vi "DriveStraight4.vi"(7 "Re-Init":bool, 9 "arguments":string[](array[string]), 10 "SensorInputData":T5, 11 "HMI to Control":T1) -> (2 "HMI to Control Out":T1, 3 "SensorInputDataOut":T5, 4 "Done":bool)   [LabVIEW 2015]
uses:
  Typedefs/SensorInputData.ctl
  Typedefs/HMI_to_Control.ctl
  Typedefs/Arm States.ctl
  Typedefs/ClawStates.ctl
  Typedefs/IntakeWheelSenseOrManual.ctl
  scriptlib/auto_data.vi
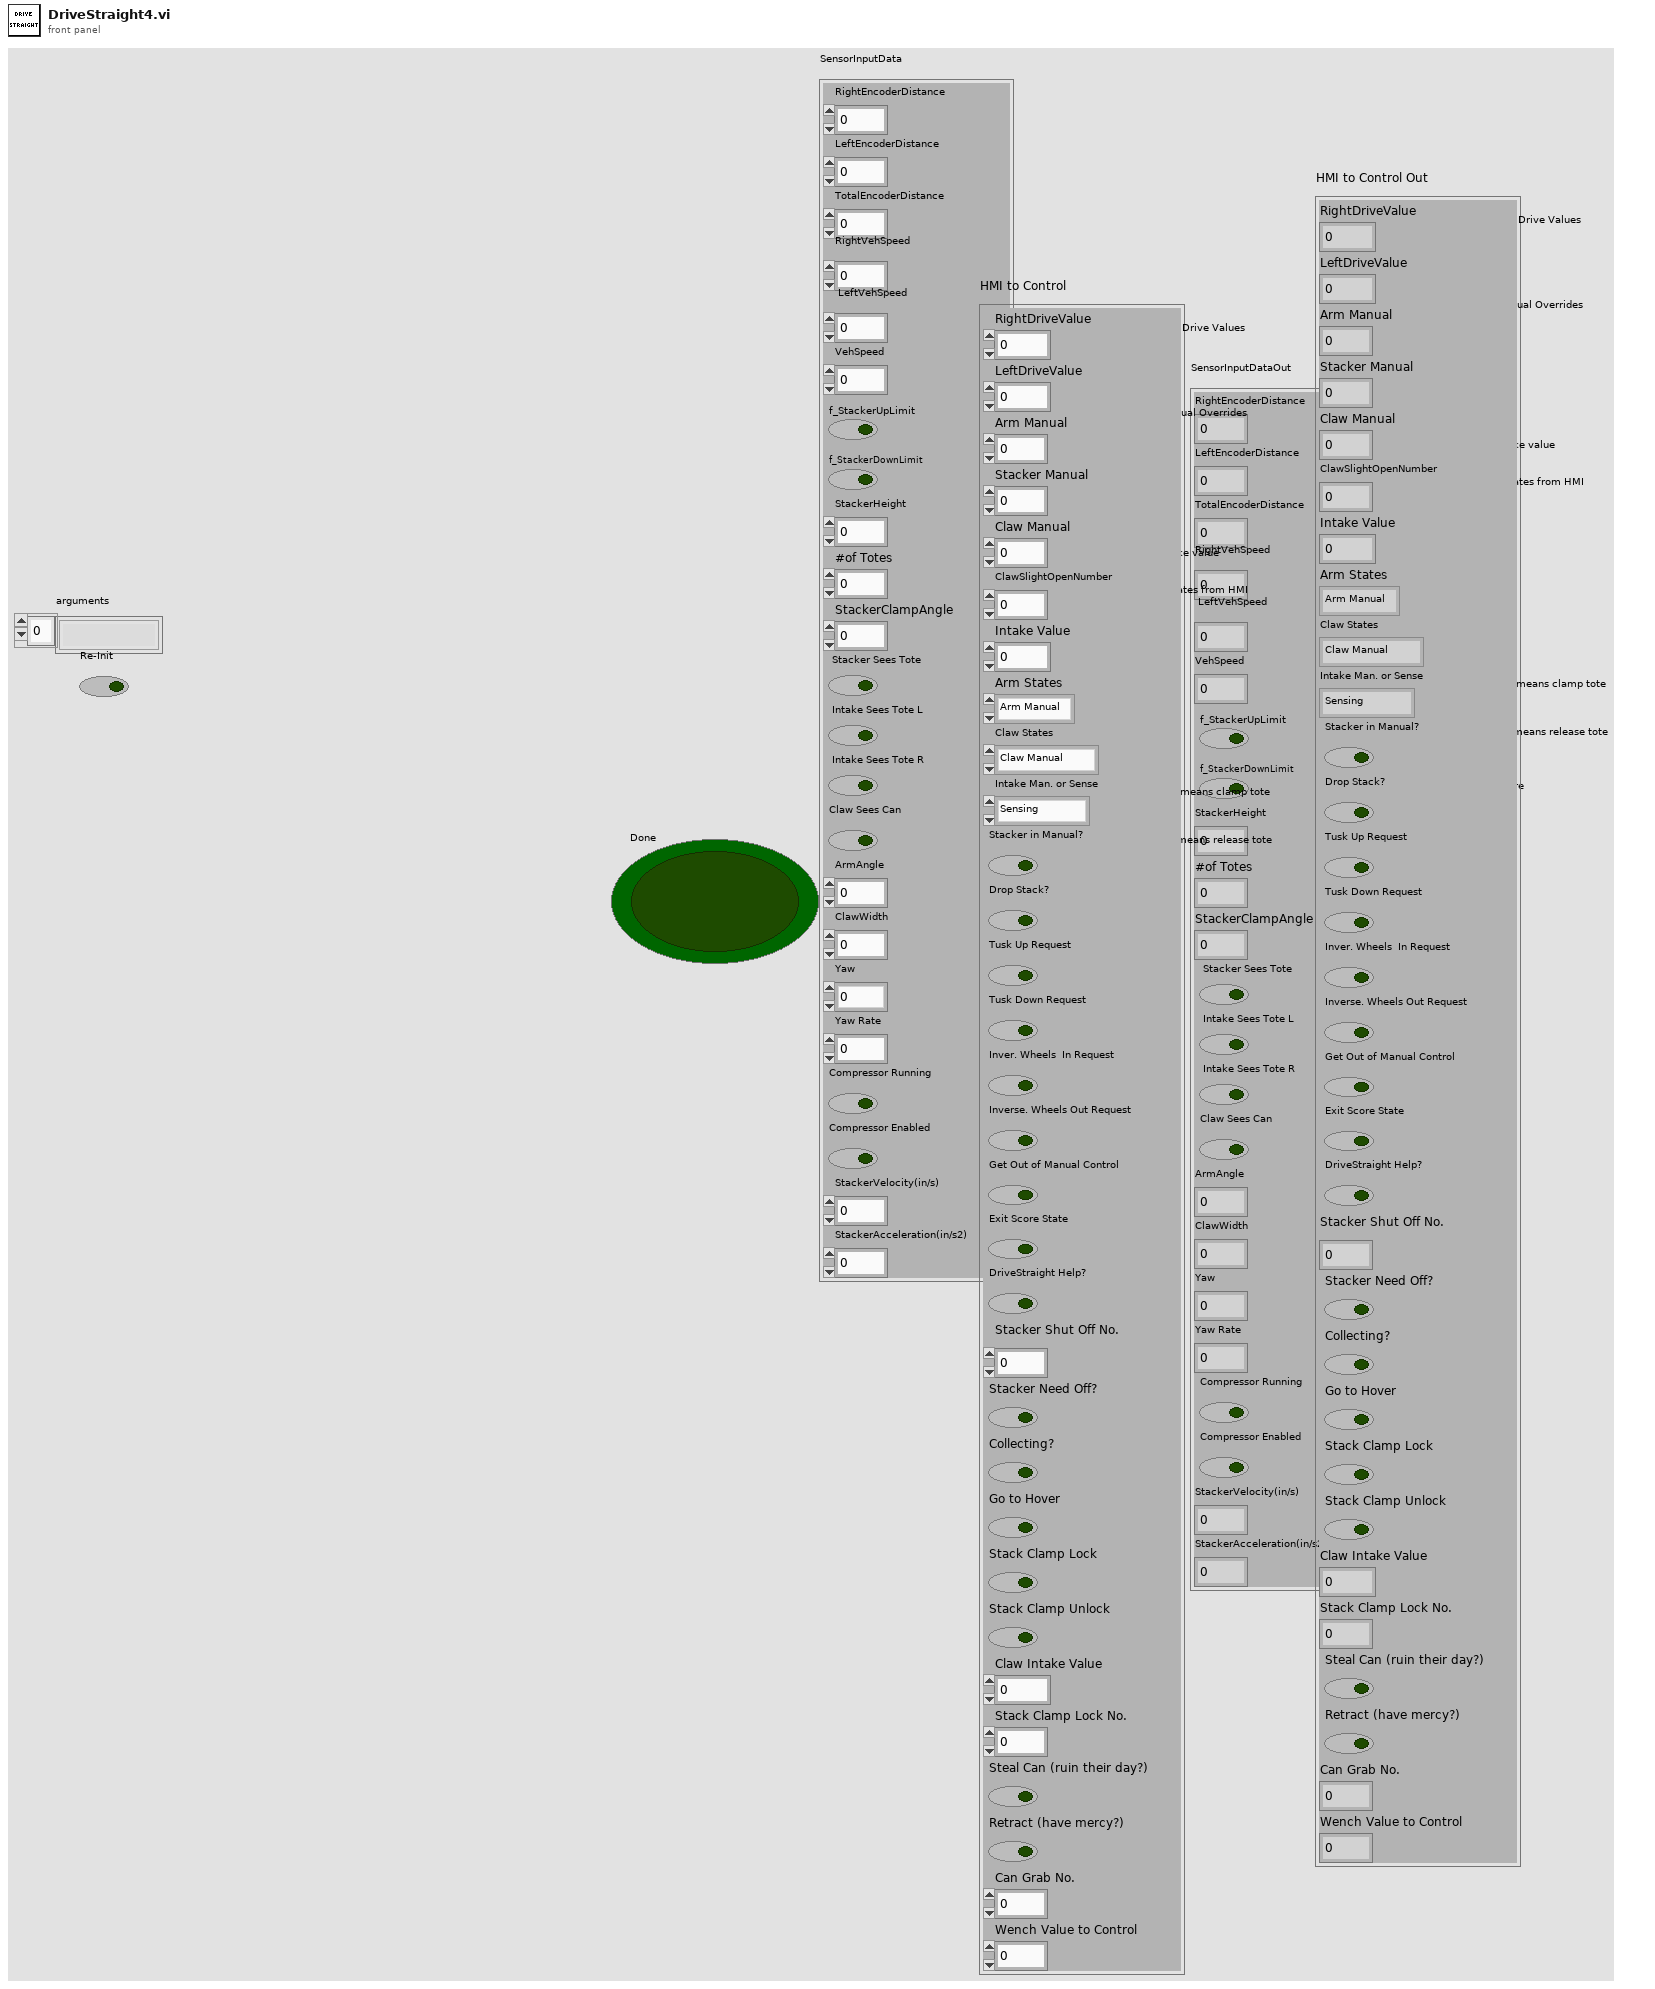
[diagram p1: front panel]
types:
  T1 = typedef "HMI_to_Control.ctl" = cluster{"RightDriveValue":dbl, "LeftDriveValue":dbl, "Arm Manual ":dbl, "Stacker Manual ":dbl, "Claw Manual ":dbl, "ClawSlightOpenNumber":i8, "Intake Value ":sgl, "Arm States":T2, "Claw States":T3, "Intake Man. or Sense":T4, "Stacker in Manual?":bool, "Drop Stack? ":bool, "Tusk Up Request":bool, "Tusk Down Request":bool, "Inver. Wheels  In Request":bool, "Inverse. Wheels Out Request ":bool, "Get Out of Manual Control":bool, "Exit Score State":bool, "DriveStraight Help?":bool, "Stacker Shut Off No.":i8, "Stacker Need Off?":bool, "Collecting?":bool, "Go to Hover":bool, "Stack Clamp Lock ":bool, "Stack Clamp Unlock ":bool, "Claw Intake Value ":sgl, "Stack Clamp Lock No. ":i8, "Steal Can (ruin their day?)":bool, "Retract (have mercy?)":bool, "Can Grab No. ":i8, "Wench Value to Control ":dbl}
  T2 = typedef "Arm States.ctl" = enum16{"Arm Manual ", "Ground", "Step", "1 Tote", "2 Tote", "3 Tote", "4 Tote", "5 Tote", "6 Tote", "Flip Can Arm", "Grab Can in auto", "Nudge"}
  T3 = typedef "ClawStates.ctl" = enum16{"Claw Manual ", "Claw Open", "Claw Closed", "Claw Slight Open", "Flip Can"}
  T4 = typedef "IntakeWheelSenseOrManual.ctl" = enum16{"Sensing", "Manual "}
  T5 = typedef "SensorInputData.ctl" = cluster{"RightEncoderDistance":dbl, "LeftEncoderDistance":dbl, "TotalEncoderDistance":dbl, "RightVehSpeed":dbl, "LeftVehSpeed":dbl, "VehSpeed":dbl, "f_StackerUpLimit":bool, "f_StackerDownLimit":bool, "StackerHeight":dbl, "#of Totes":u8, "StackerClampAngle":dbl, "Stacker Sees Tote":bool, "Intake Sees Tote L":bool, "Intake Sees Tote R":bool, "Claw Sees Can":bool, "ArmAngle":dbl, "ClawWidth":dbl, "Yaw":dbl, "Yaw Rate":dbl, "Compressor Running":bool, "Compressor Enabled":bool, "StackerVelocity(in/s)":dbl, "StackerAcceleration(in/s2)":dbl}
  T6 = cluster{"LeftEncoderDistance":dbl, "RightEncoderDistance":dbl}
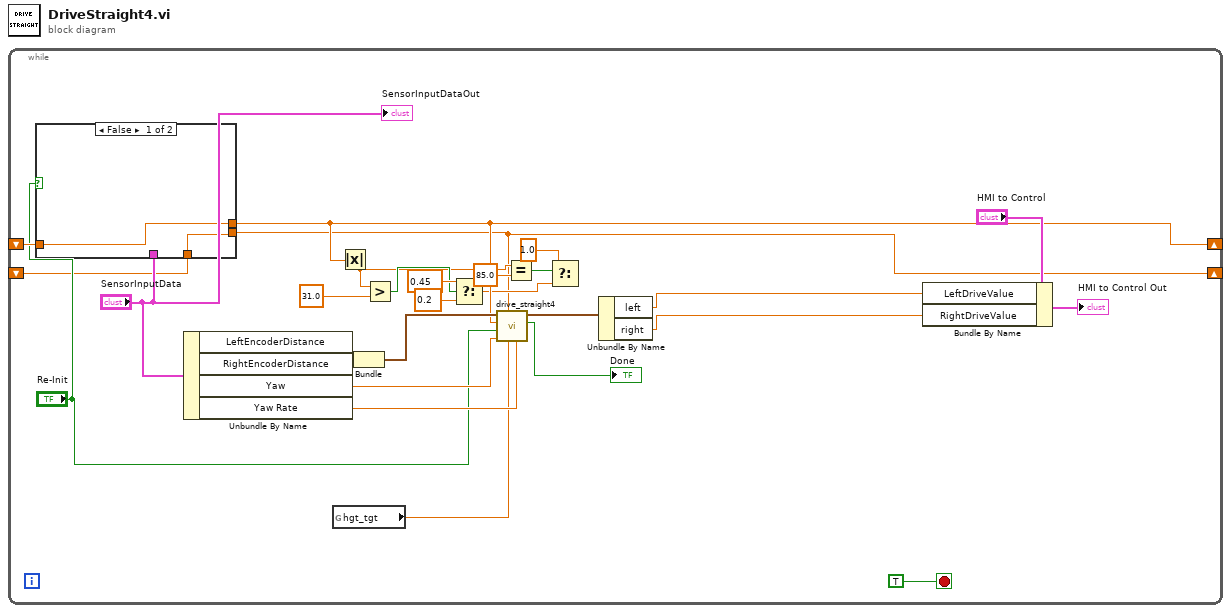
[diagram p0: block diagram]
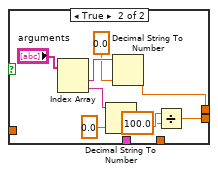
[diagram p2: hidden frame]
diagram:
  n1 = while {
    shift-right: [w8] -> _
    shift-left: _ -> [w24]
    shift-right: [w2] -> _
    shift-left: _ -> [w1]
    stop <- TRUE stop-if-true
    n2 = case shown="False" "Re-Init" {
      tunnel: [w30 w37] -> w8
      tunnel: "SensorInputData" -> [_ _]
      tunnel: w24 -> [w30 _]
      tunnel: [w29 w31] -> w2
      tunnel: w1 -> [w29 _]
      frame False {
      }
      frame True {
        n3 = Index Array(array="arguments") -> (element #1=w38:string, element #2=w35:string)  [unwired: 2 in]
        n4 = Decimal String To Number(string=w35, default (0L)=0.0) -> (number=w33:dbl)  [unwired: 1 in, 1 out]
        n5 = Decimal String To Number(string=w38, default (0L)=0.0) -> (number=w37:dbl)  [unwired: 1 in, 1 out]
        n6 = Divide(x=w33, y=100.0) -> (x/y=w31:dbl)
      }
    }
    n7 = Unbundle By Name("SensorInputData") -> ("LeftEncoderDistance"=w23:dbl, "RightEncoderDistance"=w22:dbl, "Yaw"=w20:dbl, "Yaw Rate"=w19:dbl)
    n8 = global read "auto_data.vi" "hgt_tgt"() -> (w10:dbl)
    n9 = Absolute Value(x=w8) -> (abs(x)=w7:dbl)
    n10 = Bundle("LeftEncoderDistance"=w23, "RightEncoderDistance"=w22) -> (w21:T6)  [unwired: 1 in]
    n11 = Greater?(x=w7, y=31.0 ("S")) -> (0:w11:bool)
    n12 = Select(t=0.45, s=w11, f=0.2) -> (s? t:f=w3:dbl)
    n13 = call "drive_straight4.vi"("YawRate_Meas"=w19, "YawTgt"=w10, "Output Power Limit"=w2, "YawMeas"=w20, "Init"="Re-Init", "DistanceTgt"=w8, "EncoderVal"=w21) -> ("Done"=→"Done":bool, "MotorCmdOut"=w17:cluster{"left":dbl, "right":dbl})  [unwired: 3 in]
    n14 = Equal?(x=w7, y=85.0) -> (x = y?=w5:bool)
    n15 = Select(t=1.0, s=w5, f=w3) -> ()  [unwired: 1 out]
    n16 = Unbundle By Name(w17) -> ("left"=w15:dbl, "right"=w16:dbl)
    n17 = Bundle By Name(cluster="HMI to Control", "LeftDriveValue"=w15, "RightDriveValue"=w16) -> (→"HMI to Control Out":T1)
    "SensorInputDataOut" <- "SensorInputData"
  }
